vi "Get_criterion.vi"(8 "error in":errorcluster, 11 "WLAN Test Text Input":string="TX_VERIFY_EVM 5320 OFDM6 20M TX2") -> (0 "error out":errorcluster, 2 "BT_Range":T2, 3 "WLAN_Range":T1)   [LabVIEW 2012]
uses:
  <vilib>/Utility/file.llb/Read From Spreadsheet File (string).vi
panel:
  in  "MHz 2":i16=20
  out "Violation%":string
  out "row 2":i32
  out "time spend(ms)":u32
  out "Test iItem":string
  out "row":i32
  out "mode number":dbl
  out "Mode":enum16{"OFDM", "DSSS", "MCS"}(ring)
  out "column":i32
  out "Numeric":i32
  in  "MHz":i16=20
  in  "Mode string in":string="MCS7"
  out "frequency string":string
  in  "Frequency":dbl=2412000000.0 format="%#_6p"
  out "Classified Array":string[][][](array[string])
  out "Criterion array":string[][](array[string])
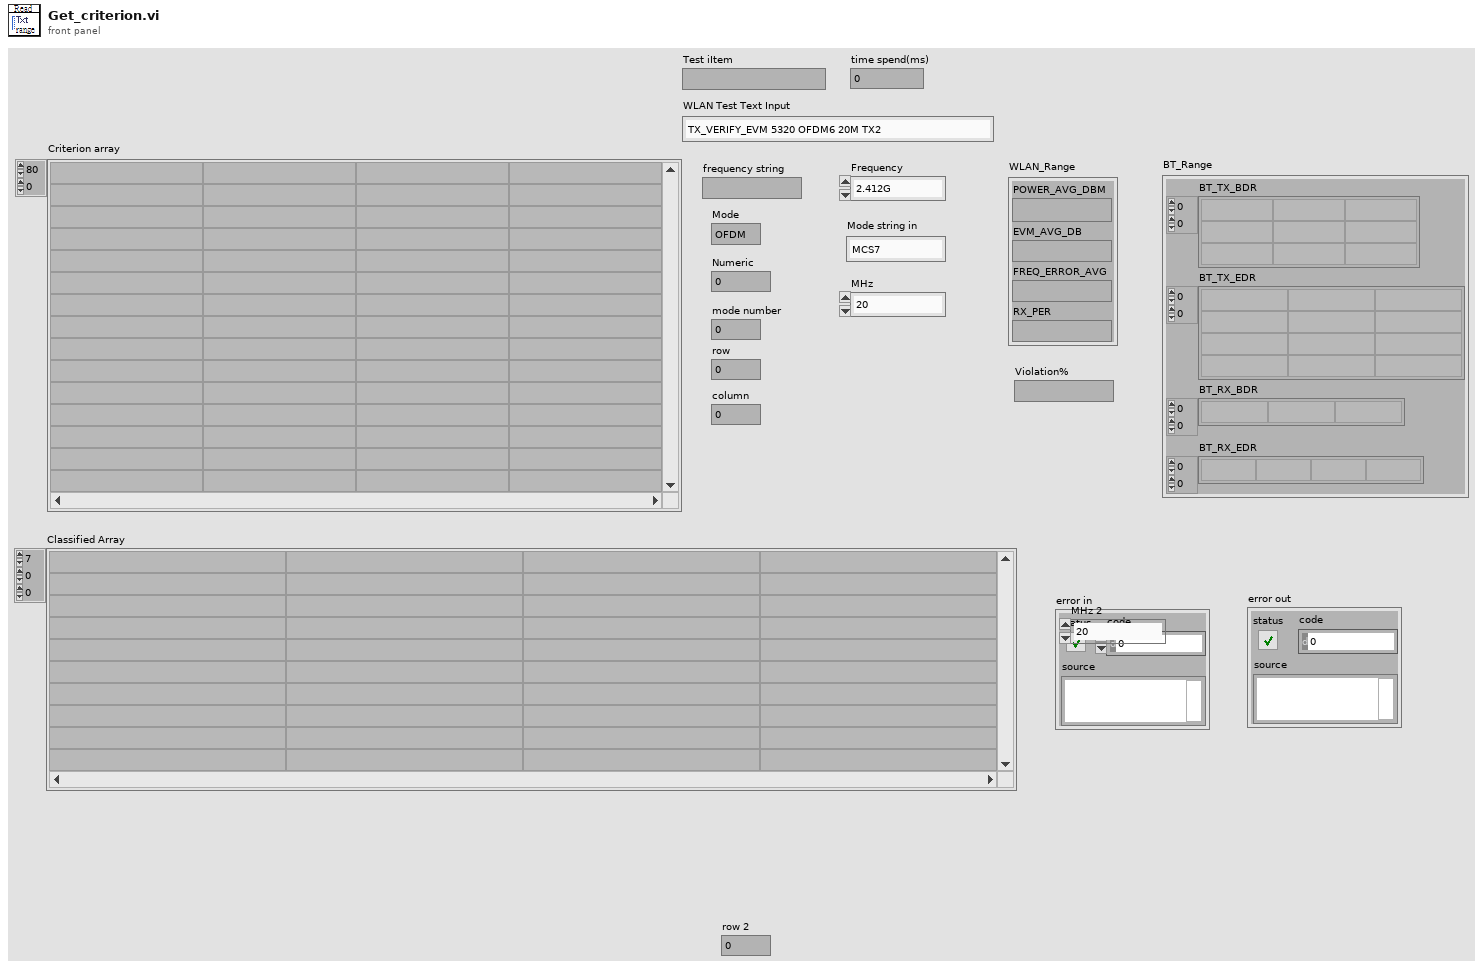
[diagram p1: front panel]
types:
  T1 = cluster{"POWER_AVG_DBM":string, "EVM_AVG_DB":string, "FREQ_ERROR_AVG":string, "RX_PER":string}
  T2 = cluster{"BT_TX_BDR":string[][], "BT_TX_EDR":string[][], "BT_RX_BDR":string[][], "BT_RX_EDR":string[][]}
  T3 = enum32{"invalid app kind", "Development System", "Run Time System", "Student Edition", "Embedded LabVIEW", "Evaluation", "Custom"}
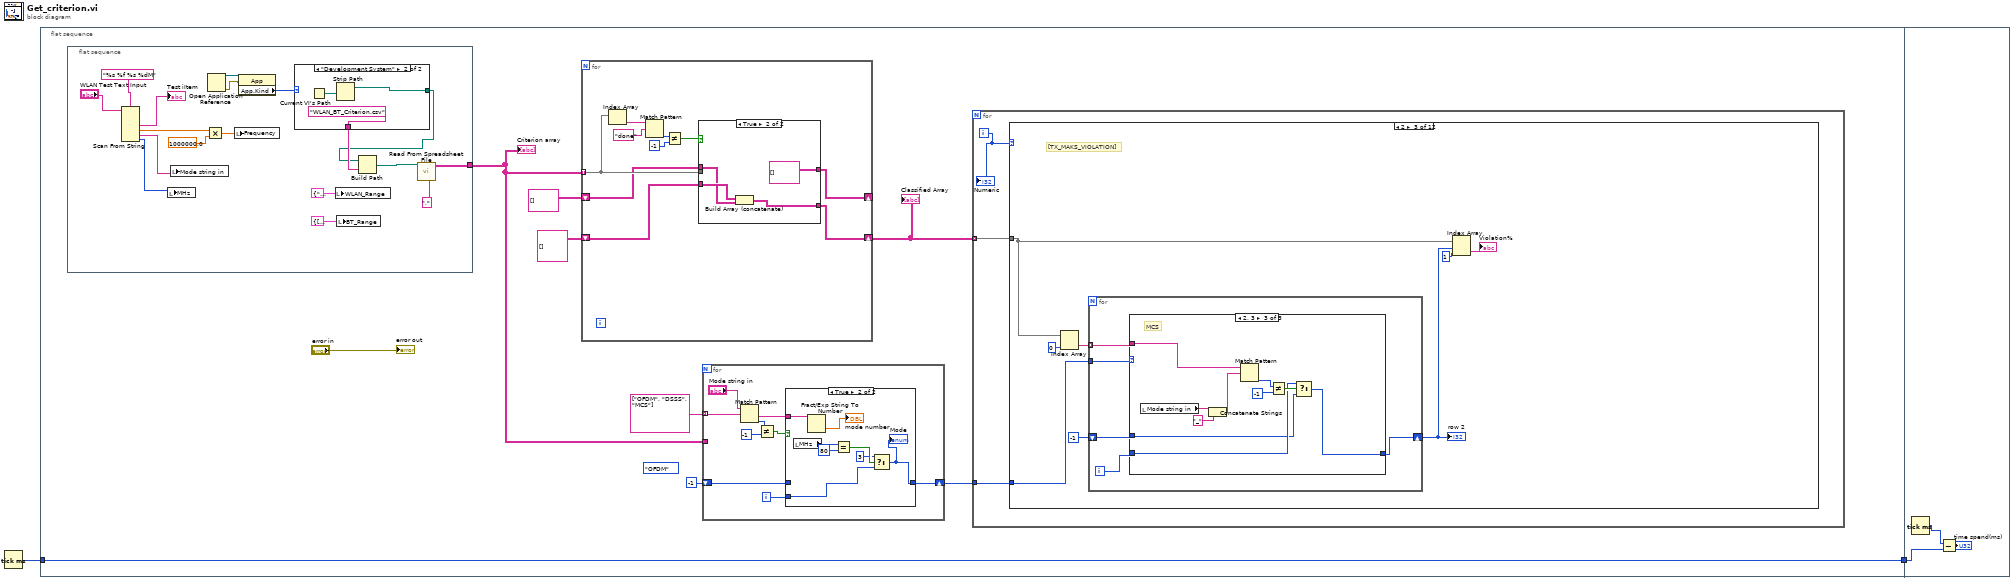
[diagram p0: block diagram]
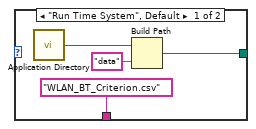
[diagram p2: hidden frame]
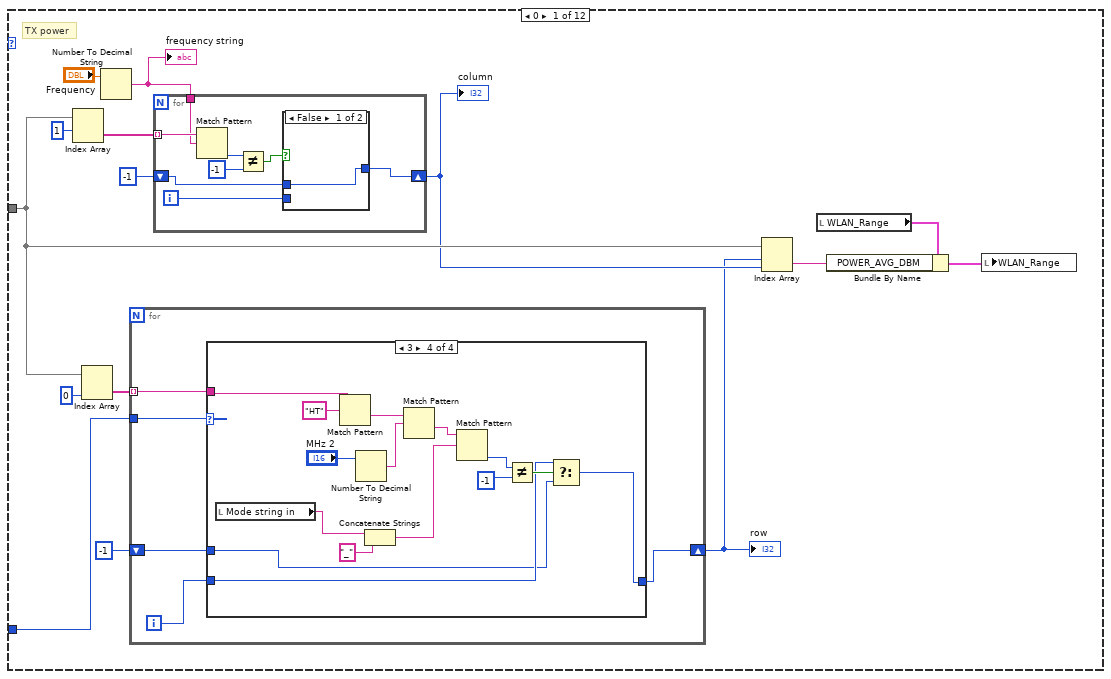
[diagram p4: hidden frame]
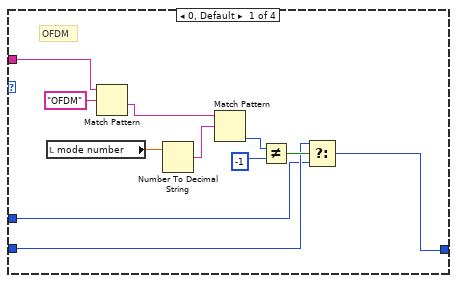
[diagram p5: hidden frame]
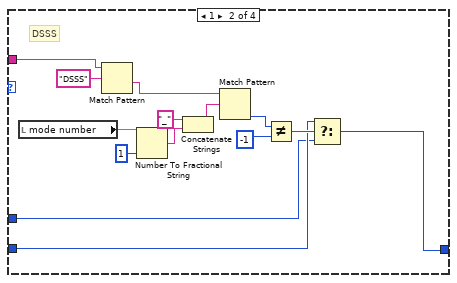
[diagram p6: hidden frame]
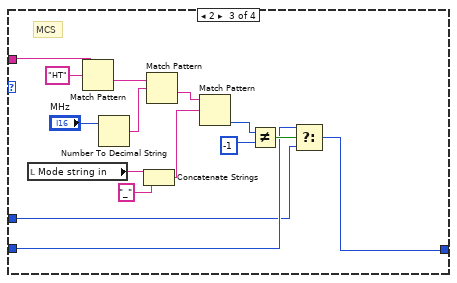
[diagram p7: hidden frame]
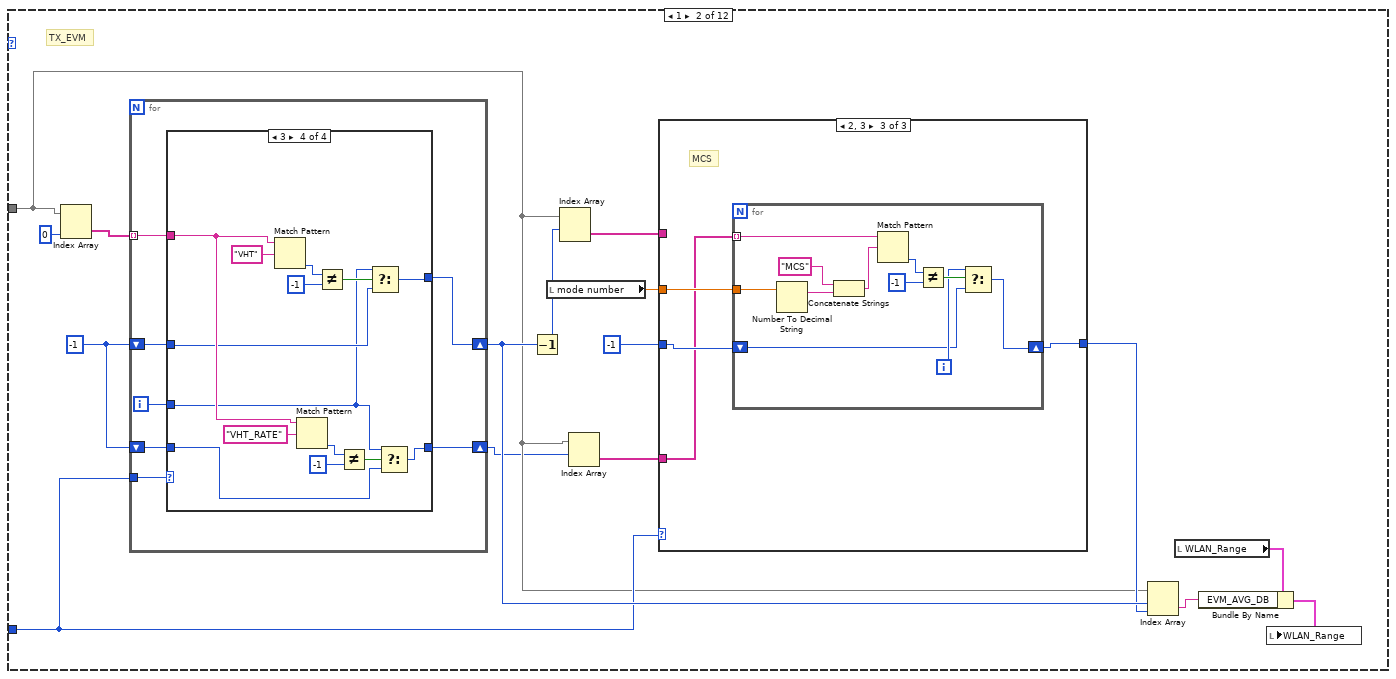
[diagram p9: hidden frame]
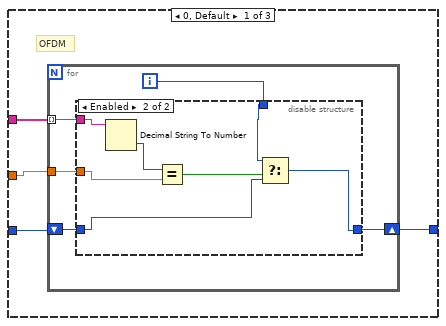
[diagram p10: hidden frame]
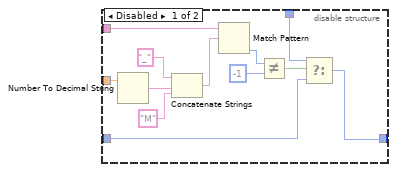
[diagram p11: hidden frame]
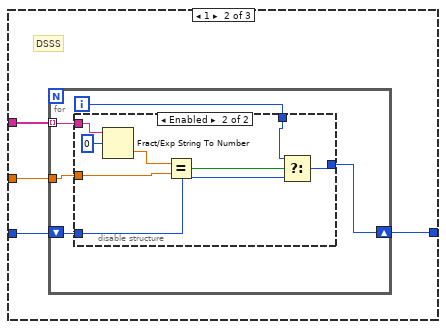
[diagram p12: hidden frame]
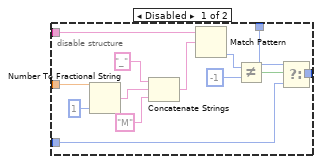
[diagram p13: hidden frame]
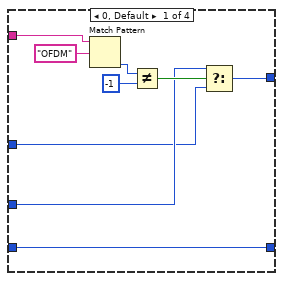
[diagram p14: hidden frame]
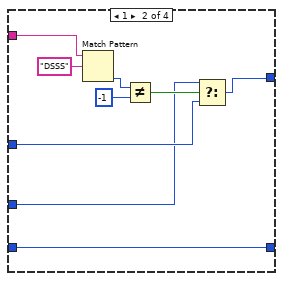
[diagram p15: hidden frame]
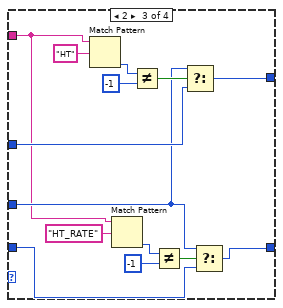
[diagram p16: hidden frame]
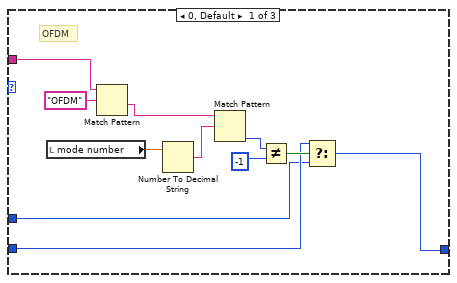
[diagram p17: hidden frame]
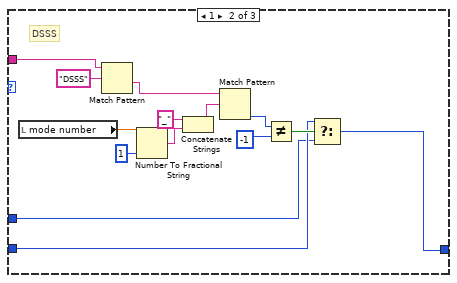
[diagram p18: hidden frame]
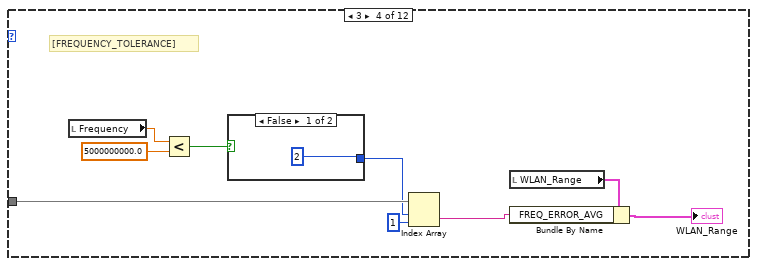
[diagram p19: hidden frame]
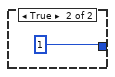
[diagram p20: hidden frame]
diagram:
  n1 = Tick Count (ms)() -> (millisecond timer value=w2:u32)
  n2 = flat-sequence {
    tunnel: w2 -> [w4]
    tunnel: [w4] -> w1
    tunnel: w1 -> [w502]
    frame #0 {
      (unwired) enum16{"OFDM", "DSSS", "MCS"}."OFDM"
      n3 = flat-sequence {
        tunnel: [w28] -> w3
        frame #0 {
          n4 = Scan From String(format string="%s %f %s %dM", input string="WLAN Test Text Input") -> (output 1=→"Test iItem":string, output 2=w21:dbl, output 3=w18:string, output 4=w17:i32)  [unwired: 6 in, 3 out]
          n5 = local write "MHz"(w17) -> ()
          n6 = local write "Mode string in"(w18) -> ()
          n7 = Multiply(x=w21, y=1000000.0) -> (x*y=w19:dbl)
          n8 = Open Application Reference() -> (0:w15:errorcluster, 3:w16:refnum<vi>)  [unwired: 4 in]
          n9 = local write "Frequency"(w19) -> ()
          n10 = property class="App"(reference=w16, error in=w15) -> ("App.Kind"=w14:T3)  [unwired: 2 out]
          n11 = case shown="\"Development System\"" w14 {
            tunnel: [w31 w35] -> w12
            tunnel: ["WLAN_BT_Criterion.csv" ("name or relative path") "WLAN_BT_Criterion.csv" ("name or relative path")] -> w13
            frame "Run Time System", Default {
              n12 = call <vilib>:"Application Directory.vi"() -> ("Application Directory"=w33:path)
              n13 = Build Path(base path=w33, name or relative path="data") -> (appended path=w31:path)
            }
            frame "Development System" {
              n14 = Current VI's Path() -> (path=w36:path)
              n15 = Strip Path(path=w36) -> (stripped path=w35:path)  [unwired: 1 out]
            }
          }
          n16 = local write "WLAN_Range"(T1 {"POWER_AVG_DBM"="", "EVM_AVG_DB"="", "FREQ_ERROR_AVG"="", "RX_PER"=""} ("WLAN_Range")) -> ()
          n17 = local write "BT_Range"(T2 {"BT_TX_BDR"=[], "BT_TX_EDR"=[], "BT_RX_BDR"=[], "BT_RX_EDR"=[]} ("BT_Range")) -> ()
          n18 = Build Path(base path=w12, name or relative path=w13) -> (appended path=w25:path)
          n19 = call-poly <vilib>:"Read From Spreadsheet File.vi"("delimiter (\\t)"="," ("delimiter (\\t)"), "file path (dialog if empty)"=w25) -> ("all rows"=w28:string[][])  [unwired: 5 in, 4 out]
        }
      }
      n20 = for {
        tunnel: w3 -> [w491] mode=indexing
        shift-right: [w489] -> _
        shift-left: string[][] [] -> [w490]
        shift-right: [w487] -> w6
        shift-left: string[][][] [] -> [w488]
        n21 = Index Array(array=w491) -> (element=w486:string)  [unwired: 1 in]
        n22 = Match Pattern(string=w486, regular expression="done") -> (offset past match=w484:i32)  [unwired: 1 in, 3 out]
        n23 = Not Equal?(x=w484, y=-1) -> (x != y?=w482:bool)
        n24 = case shown="True" w482 {
          tunnel: w490 -> [w495 w497]
          tunnel: w491 -> [w494 _]
          tunnel: [w493 string[][] []] -> w489
          tunnel: w488 -> [w492 w498]
          tunnel: [w492 w496] -> w487
          frame False {
            n25 = Build Array (concatenate)(w495, w494) -> (w493:string[][])
          }
          frame True {
            n26 = Build Array (concatenate)(w498, w497) -> (w496:string[][][])
          }
        }
      }
      "Classified Array" <- w6
      n27 = for {
        tunnel: string[] ["OFDM", "DSSS", "MCS"] -> [w44] mode=indexing
        shift-right: [w38] -> w8
        shift-left: -1 -> [w37]
        tunnel: w3 -> [_]
        i -> [w40]
        n28 = Match Pattern(string="Mode string in", regular expression=w44) -> (after substring=w39:string, offset past match=w43:i32)  [unwired: 1 in, 2 out]
        n29 = Not Equal?(x=w43, y=-1) -> (x != y?=w41:bool)
        n30 = case shown="True" w41 {
          tunnel: w40 -> [_ w48]
          tunnel: w39 -> [_ w54]
          tunnel: [w46 w47] -> w38
          tunnel: w37 -> [w46 _]
          frame False {
          }
          frame True {
            n31 = local read "MHz"() -> (w52:i16)
            n32 = Fract/Exp String To Number(string=w54) -> (number=→"mode number":dbl)  [unwired: 3 in, 1 out]
            n33 = Equal?(x=w52, y=i16 80) -> (x = y?=w50:bool)
            n34 = Select(t=3, s=w50, f=w48) -> (s? t:f=w47:i32)
            "Mode" <- w47
          }
        }
      }
      n35 = for {
        tunnel: w6 -> [w56] mode=indexing
        tunnel: w8 -> [w55]
        i -> [w57]
        n36 = case shown="2" w57 {
          tunnel: w56 -> [w63 w148 w288 w338 w349 _ _ w390 w413 w437 w461 _]
          tunnel: w55 -> [w65 w152 w289 _ w351 _ _ _ _ _ _ _]
          frame 0 {
            # "TX power"
            n37 = Index Array(array=w63, index (row)=1) -> (element=w70:string[])  [unwired: 1 in]
            n38 = Index Array(array=w63, index (col)=0) -> (element=w66:string[])  [unwired: 1 in]
            n39 = Number To Decimal String(number="Frequency") -> (decimal integer string=w69:string)  [unwired: 1 in]
            "frequency string" <- w69
            n40 = for {
              tunnel: w66 -> [w75] mode=indexing
              tunnel: w65 -> [w77]
              shift-right: [w74] -> w61
              shift-left: -1 -> [w73]
              i -> [w76]
              n41 = case shown="3" w77 {
                tunnel: w76 -> [w80 w94 w105 w120]
                tunnel: w75 -> [w87 w97 w116 w124]
                tunnel: [w79 w92 w103 w118] -> w74
                tunnel: w73 -> [w78 w93 w104 w119]
                frame 0, Default {
                  # "OFDM"
                  n42 = local read "mode number"() -> (w85:dbl)
                  n43 = Match Pattern(string=w87, regular expression="OFDM") -> (after substring=w86:string)  [unwired: 1 in, 3 out]
                  n44 = Number To Decimal String(number=w85) -> (decimal integer string=w84:string)  [unwired: 1 in]
                  n45 = Match Pattern(string=w86, regular expression=w84) -> (offset past match=w83:i32)  [unwired: 1 in, 3 out]
                  n46 = Not Equal?(x=w83, y=-1) -> (x != y?=w81:bool)
                  n47 = Select(t=w80, s=w81, f=w78) -> (s? t:f=w79:i32)
                }
                frame 1 {
                  # "DSSS"
                  n48 = local read "mode number"() -> (w96:dbl)
                  n49 = Match Pattern(string=w97, regular expression="DSSS") -> (after substring=w101:string)  [unwired: 1 in, 3 out]
                  n50 = Number To Fractional String(number=w96, precision (6)=i16 1) -> (F-format string=w90:string)  [unwired: 2 in]
                  n51 = Concatenate Strings("_" ("string"), w90) -> (w91:string)
                  n52 = Match Pattern(string=w101, regular expression=w91) -> (offset past match=w100:i32)  [unwired: 1 in, 3 out]
                  n53 = Not Equal?(x=w100, y=-1) -> (x != y?=w98:bool)
                  n54 = Select(t=w94, s=w98, f=w93) -> (s? t:f=w92:i32)
                }
                frame 2 {
                  # "MCS"
                  n55 = local read "Mode string in"() -> (w111:string)
                  n56 = Match Pattern(string=w116, regular expression="HT") -> (after substring=w114:string)  [unwired: 1 in, 3 out]
                  n57 = Number To Decimal String(number="MHz") -> (decimal integer string=w113:string)  [unwired: 1 in]
                  n58 = Concatenate Strings(w111, "_" ("string")) -> (w109:string)
                  n59 = Match Pattern(string=w114, regular expression=w113) -> (after substring=w112:string)  [unwired: 1 in, 3 out]
                  n60 = Match Pattern(string=w112, regular expression=w109) -> (offset past match=w107:i32)  [unwired: 1 in, 3 out]
                  n61 = Not Equal?(x=w107, y=-1) -> (x != y?=w106:bool)
                  n62 = Select(t=w105, s=w106, f=w104) -> (s? t:f=w103:i32)
                }
                frame 3 {
                  n63 = local read "Mode string in"() -> (w122:string)
                  n64 = Match Pattern(string=w124, regular expression="HT") -> (after substring=w130:string)  [unwired: 1 in, 3 out]
                  n65 = Number To Decimal String(number="MHz 2") -> (decimal integer string=w129:string)  [unwired: 1 in]
                  n66 = Concatenate Strings(w122, "_" ("string")) -> (w121:string)
                  n67 = Match Pattern(string=w130, regular expression=w129) -> (after substring=w128:string)  [unwired: 1 in, 3 out]
                  n68 = Match Pattern(string=w128, regular expression=w121) -> (offset past match=w126:i32)  [unwired: 1 in, 3 out]
                  n69 = Not Equal?(x=w126, y=-1) -> (x != y?=w125:bool)
                  n70 = Select(t=w120, s=w125, f=w119) -> (s? t:f=w118:i32)
                }
              }
            }
            "row" <- w61
            n71 = for {
              tunnel: w70 -> [w140] mode=indexing
              tunnel: w69 -> [w139]
              shift-right: [w134] -> w62
              shift-left: -1 -> [w133]
              i -> [w135]
              n72 = Match Pattern(string=w140, regular expression=w139) -> (offset past match=w138:i32)  [unwired: 1 in, 3 out]
              n73 = Not Equal?(x=w138, y=-1) -> (x != y?=w136:bool)
              n74 = case shown="False" w136 {
                tunnel: w135 -> [_ w142]
                tunnel: [w141 w142] -> w134
                tunnel: w133 -> [w141 _]
                frame False {
                }
                frame True {
                }
              }
            }
            "column" <- w62
            n75 = Index Array(array=w63, index (row)=w61, index (col)=w62) -> (element=w59:string)
            n76 = local read "WLAN_Range"() -> (w58:T1)
            n77 = Bundle By Name(cluster=w58, "POWER_AVG_DBM"=w59) -> (w60:T1)
            n78 = local write "WLAN_Range"(w60) -> ()
          }
          frame 1 {
            w149 = -1
            # "TX_EVM"
            n79 = Index Array(array=w148, index (col)=0) -> (element=w157:string[])  [unwired: 1 in]
            n80 = for {
              tunnel: w157 -> [w237] mode=indexing
              tunnel: w152 -> [w238]
              shift-right: [w234] -> w154
              shift-left: w149 -> [w235]
              shift-right: [w232] -> w147
              shift-left: w149 -> [w233]
              i -> [w236]
              n81 = case shown="3" w238 {
                tunnel: w237 -> [w246 w253 w257 w276]
                tunnel: w236 -> [w242 w250 w260 w274]
                tunnel: w235 -> [w241 w251 w266 w275]
                tunnel: [w240 w249 w265 w272] -> w234
                tunnel: w233 -> [w239 w248 w259 w273]
                tunnel: [w239 w248 w258 w271] -> w232
                frame 0, Default {
                  n82 = Match Pattern(string=w246, regular expression="OFDM") -> (offset past match=w245:i32)  [unwired: 1 in, 3 out]
                  n83 = Not Equal?(x=w245, y=-1) -> (x != y?=w243:bool)
                  n84 = Select(t=w242, s=w243, f=w241) -> (s? t:f=w240:i32)
                }
                frame 1 {
                  n85 = Match Pattern(string=w253, regular expression="DSSS") -> (offset past match=w256:i32)  [unwired: 1 in, 3 out]
                  n86 = Not Equal?(x=w256, y=-1) -> (x != y?=w254:bool)
                  n87 = Select(t=w250, s=w254, f=w251) -> (s? t:f=w249:i32)
                }
                frame 2 {
                  n88 = Match Pattern(string=w257, regular expression="HT") -> (offset past match=w269:i32)  [unwired: 1 in, 3 out]
                  n89 = Match Pattern(string=w257, regular expression="HT_RATE") -> (offset past match=w262:i32)  [unwired: 1 in, 3 out]
                  n90 = Not Equal?(x=w269, y=-1) -> (x != y?=w267:bool)
                  n91 = Not Equal?(x=w262, y=-1) -> (x != y?=w264:bool)
                  n92 = Select(t=w260, s=w267, f=w266) -> (s? t:f=w265:i32)
                  n93 = Select(t=w260, s=w264, f=w259) -> (s? t:f=w258:i32)
                }
                frame 3 {
                  n94 = Match Pattern(string=w276, regular expression="VHT") -> (offset past match=w283:i32)  [unwired: 1 in, 3 out]
                  n95 = Match Pattern(string=w276, regular expression="VHT_RATE") -> (offset past match=w278:i32)  [unwired: 1 in, 3 out]
                  n96 = Not Equal?(x=w283, y=-1) -> (x != y?=w281:bool)
                  n97 = Not Equal?(x=w278, y=-1) -> (x != y?=w280:bool)
                  n98 = Select(t=w274, s=w281, f=w275) -> (s? t:f=w272:i32)
                  n99 = Select(t=w274, s=w280, f=w273) -> (s? t:f=w271:i32)
                }
              }
            }
            n100 = Decrement(x=w154) -> (x-1=w156:i32)
            n101 = local read "mode number"() -> (w151:dbl)
            n102 = Index Array(array=w148, index (row)=w156) -> (element=w155:string[])  [unwired: 1 in]
            n103 = Index Array(array=w148, index (row)=w147) -> (element=w146:string[])  [unwired: 1 in]
            n104 = case shown="2, 3" w152 {
              tunnel: w155 -> [w162 w190 _]
              tunnel: [w161 w189 w217] -> w153
              tunnel: w151 -> [w160 w188 w219]
              tunnel: -1 -> [w159 w187 w220]
              tunnel: w146 -> [_ _ w218]
              frame 0, Default {
                # "OFDM"
                n105 = for {
                  tunnel: w162 -> [w167] mode=indexing
                  shift-right: [w164] -> w161
                  shift-left: w159 -> [w165]
                  tunnel: w160 -> [w163]
                  i -> [w166]
                  n106 = disable-structure shown="Enabled" {
                    disable-tunnel: w167 -> [w179 w186]
                    disable-tunnel: w166 -> [w178 w182]
                    disable-tunnel: w165 -> [w177 w181]
                    disable-tunnel: [w176 w180] -> w164
                    disable-tunnel: w163 -> [w175 w184]
                    frame Disabled {
                      n107 = Number To Decimal String(number=w175) -> (decimal integer string=w171:string)  [unwired: 1 in]
                      n108 = Concatenate Strings("_" ("string"), w171, "M" ("string")) -> (w168:string)
                      n109 = Match Pattern(string=w179, regular expression=w168) -> (offset past match=w173:i32)  [unwired: 1 in, 3 out]
                      n110 = Not Equal?(x=w173, y=-1) -> (x != y?=w172:bool)
                      n111 = Select(t=w178, s=w172, f=w177) -> (s? t:f=w176:i32)
                    }
                    frame Enabled {
                      n112 = Decimal String To Number(string=w186) -> (number=w185:i32)  [unwired: 2 in, 1 out]
                      n113 = Equal?(x=w185, y=w184) -> (x = y?=w183:bool)
                      n114 = Select(t=w182, s=w183, f=w181) -> (s? t:f=w180:i32)
                    }
                  }
                }
              }
              frame 1 {
                # "DSSS"
                n115 = for {
                  tunnel: w190 -> [w195] mode=indexing
                  shift-right: [w192] -> w189
                  shift-left: w187 -> [w193]
                  tunnel: w188 -> [w191]
                  i -> [w194]
                  n116 = disable-structure shown="Enabled" {
                    disable-tunnel: w195 -> [w208 w216]
                    disable-tunnel: w194 -> [w204 w212]
                    disable-tunnel: w193 -> [w203 w211]
                    disable-tunnel: [w202 w210] -> w192
                    disable-tunnel: w191 -> [w196 w214]
                    frame Disabled {
                      n117 = Number To Fractional String(number=w196, precision (6)=i16 1) -> (F-format string=w197:string)  [unwired: 2 in]
                      n118 = Concatenate Strings("_" ("string"), w197, "M" ("string")) -> (w199:string)
                      n119 = Match Pattern(string=w208, regular expression=w199) -> (offset past match=w206:i32)  [unwired: 1 in, 3 out]
                      n120 = Not Equal?(x=w206, y=-1) -> (x != y?=w205:bool)
                      n121 = Select(t=w204, s=w205, f=w203) -> (s? t:f=w202:i32)
                    }
                    frame Enabled {
                      n122 = Fract/Exp String To Number(string=w216, offset=0) -> (number=w215:dbl)  [unwired: 2 in, 1 out]
                      n123 = Equal?(x=w215, y=w214) -> (x = y?=w213:bool)
                      n124 = Select(t=w212, s=w213, f=w211) -> (s? t:f=w210:i32)
                    }
                  }
                }
              }
              frame 2, 3 {
                # "MCS"
                n125 = for {
                  tunnel: w218 -> [w231] mode=indexing
                  shift-right: [w225] -> w217
                  shift-left: w220 -> [w226]
                  tunnel: w219 -> [w221]
                  i -> [w227]
                  n126 = Number To Decimal String(number=w221) -> (decimal integer string=w224:string)  [unwired: 1 in]
                  n127 = Concatenate Strings("MCS" ("string"), w224) -> (w222:string)
                  n128 = Match Pattern(string=w231, regular expression=w222) -> (offset past match=w229:i32)  [unwired: 1 in, 3 out]
                  n129 = Not Equal?(x=w229, y=-1) -> (x != y?=w228:bool)
                  n130 = Select(t=w227, s=w228, f=w226) -> (s? t:f=w225:i32)
                }
              }
            }
            n131 = Index Array(array=w148, index (row)=w154, index (col)=w153) -> (element=w145:string)
            n132 = local read "WLAN_Range"() -> (w143:T1)
            n133 = Bundle By Name(cluster=w143, "EVM_AVG_DB"=w145) -> (w144:T1)
            n134 = local write "WLAN_Range"(w144) -> ()
          }
          frame 2 {
            # "[TX_MAKS_VIOLATION]"
            n135 = Index Array(array=w288, index (col)=0) -> (element=w291:string[])  [unwired: 1 in]
            n136 = for {
              tunnel: w291 -> [w296] mode=indexing
              tunnel: w289 -> [w295]
              shift-right: [w297] -> w287
              shift-left: -1 -> [w294]
              i -> [w293]
              n137 = case shown="2, 3" w295 {
                tunnel: w293 -> [w300 w314 w326]
                tunnel: w296 -> [w307 w317 w323]
                tunnel: [w299 w312 w324] -> w297
                tunnel: w294 -> [w298 w313 w325]
                frame 0, Default {
                  # "OFDM"
                  n138 = local read "mode number"() -> (w305:dbl)
                  n139 = Match Pattern(string=w307, regular expression="OFDM") -> (after substring=w306:string)  [unwired: 1 in, 3 out]
                  n140 = Number To Decimal String(number=w305) -> (decimal integer string=w304:string)  [unwired: 1 in]
                  n141 = Match Pattern(string=w306, regular expression=w304) -> (offset past match=w303:i32)  [unwired: 1 in, 3 out]
                  n142 = Not Equal?(x=w303, y=-1) -> (x != y?=w301:bool)
                  n143 = Select(t=w300, s=w301, f=w298) -> (s? t:f=w299:i32)
                }
                frame 1 {
                  # "DSSS"
                  n144 = local read "mode number"() -> (w316:dbl)
                  n145 = Match Pattern(string=w317, regular expression="DSSS") -> (after substring=w321:string)  [unwired: 1 in, 3 out]
                  n146 = Number To Fractional String(number=w316, precision (6)=i16 1) -> (F-format string=w310:string)  [unwired: 2 in]
                  n147 = Concatenate Strings("_" ("string"), w310) -> (w311:string)
                  n148 = Match Pattern(string=w321, regular expression=w311) -> (offset past match=w320:i32)  [unwired: 1 in, 3 out]
                  n149 = Not Equal?(x=w320, y=-1) -> (x != y?=w318:bool)
                  n150 = Select(t=w314, s=w318, f=w313) -> (s? t:f=w312:i32)
                }
                frame 2, 3 {
                  # "MCS"
                  n151 = local read "Mode string in"() -> (w332:string)
                  n152 = Concatenate Strings(w332, "_" ("string")) -> (w330:string)
                  n153 = Match Pattern(string=w323, regular expression=w330) -> (offset past match=w328:i32)  [unwired: 1 in, 3 out]
                  n154 = Not Equal?(x=w328, y=-1) -> (x != y?=w327:bool)
                  n155 = Select(t=w326, s=w327, f=w325) -> (s? t:f=w324:i32)
                }
              }
            }
            "row 2" <- w287
            n156 = Index Array(array=w288, index (row)=w287, index (col)=1 ("disabled index (col)")) -> (element=→"Violation%":string)
          }
          frame 3 {
            # "[FREQUENCY_TOLERANCE]"
            n157 = local read "Frequency"() -> (w341:dbl)
            n158 = Less?(x=w341, y=5000000000.0) -> (x < y?=w339:bool)
            n159 = case shown="False" w339 {
              tunnel: [2 1] -> w336
              frame False {
              }
              frame True {
              }
            }
            n160 = Index Array(array=w338, index (row)=w336, index (col)=1 ("disabled index (col)")) -> (element=w335:string)
            n161 = local read "WLAN_Range"() -> (w333:T1)
            n162 = Bundle By Name(cluster=w333, "FREQ_ERROR_AVG"=w335) -> (→"WLAN_Range":T1)
          }
          frame 4 {
            # "[RX_PER]"
            n163 = Index Array(array=w349, index (col)=0 ("disabled index (col)")) -> (element=w352:string[])  [unwired: 1 in]
            n164 = for {
              tunnel: w352 -> [w357] mode=indexing
              tunnel: w351 -> [w358]
              shift-right: [w354] -> w347
              shift-left: -1 ("y") -> [w356]
              i -> [w355]
              n165 = case shown="0, Default" w358 {
                tunnel: w357 -> [w366 w371 w384]
                tunnel: w356 -> [w361 w369 w377]
                tunnel: w355 -> [w360 w368 w376]
                tunnel: [w359 w367 w375] -> w354
                frame 0, Default {
                  n166 = Match Pattern(string=w366, regular expression="OFDM") -> (offset past match=w363:i32)  [unwired: 1 in, 3 out]
                  n167 = Not Equal?(x=w363, y=-1) -> (x != y?=w362:bool)
                  n168 = Select(t=w360, s=w362, f=w361) -> (s? t:f=w359:i32)
                }
                frame 1 {
                  n169 = Match Pattern(string=w371, regular expression="DSSS") -> (offset past match=w372:i32)  [unwired: 1 in, 3 out]
                  n170 = Not Equal?(x=w372, y=-1) -> (x != y?=w370:bool)
                  n171 = Select(t=w368, s=w370, f=w369) -> (s? t:f=w367:i32)
                }
                frame 2 {
                  n172 = local read "MHz"() -> (w382:i16)
                  n173 = Match Pattern(string=w384, regular expression="HT") -> (after substring=w383:string)  [unwired: 1 in, 3 out]
                  n174 = Number To Decimal String(number=w382) -> (decimal integer string=w381:string)  [unwired: 1 in]
                  n175 = Match Pattern(string=w383, regular expression=w381) -> (offset past match=w380:i32)  [unwired: 1 in, 3 out]
                  n176 = Not Equal?(x=w380, y=-1) -> (x != y?=w378:bool)
                  n177 = Select(t=w376, s=w378, f=w377) -> (s? t:f=w375:i32)
                }
              }
            }
            n178 = Index Array(array=w349, index (row)=w347, index (col)=1 ("index (row)")) -> (element=w345:string)
            n179 = local read "WLAN_Range"() -> (w344:T1)
            n180 = Bundle By Name(cluster=w344, "RX_PER"=w345) -> (w346:T1)
            n181 = local write "WLAN_Range"(w346) -> ()
          }
          frame 5 {
            # "[RX_SENSITIVITY_START_SEARCH_POW"
          }
          frame 6 {
            # "[RX_SENSITIVITY]"
          }
          frame 7 {
            # "[BT_TX_BDR]"
            n182 = for {
              tunnel: w390 -> [w398] mode=indexing
              shift-right: [w396] -> w387
              shift-left: string[][] [] -> [w397]
              w399 = ""
              n183 = Index Array(array=w398, index #1=0 ("index"), index #2=1 ("index"), index #3=2 ("index")) -> (element #1=w402:string, element #2=w401:string, element #3=w400:string)
              n184 = Not Equal?(x=w402, y=w399) -> (x != y?=w394:bool)
              n185 = Not Equal?(x=w401, y=w399) -> (x != y?=w392:bool)
              n186 = Not Equal?(x=w400, y=w399) -> (x != y?=w393:bool)
              n187 = Or(x=w392, y=w393) -> (x .or. y?=w391:bool)
              n188 = And(x=w394, y=w391) -> (x .and. y?=w395:bool)
              n189 = case shown="True" w395 {
                tunnel: w398 -> [_ w408]
                tunnel: w397 -> [w406 w409]
                tunnel: [w406 w407] -> w396
                frame False {
                }
                frame True {
                  n190 = Build Array (concatenate)(w409, w408) -> (w407:string[][])
                }
              }
            }
            n191 = local read "BT_Range"() -> (w386:T2)
            n192 = Bundle By Name(cluster=w386, "BT_TX_BDR"=w387) -> (w388:T2)
            n193 = local write "BT_Range"(w388) -> ()
          }
          frame 8 {
            # "[BT_TX_EDR]"
            n194 = for {
              tunnel: w413 -> [w422] mode=indexing
              shift-right: [w420] -> w411
              shift-left: string[][] [] -> [w421]
              w423 = ""
              n195 = Index Array(array=w422, index #1=0 ("index"), index #2=1 ("index"), index #3=2 ("index")) -> (element #1=w426:string, element #2=w425:string, element #3=w424:string)
              n196 = Not Equal?(x=w426, y=w423) -> (x != y?=w418:bool)
              n197 = Not Equal?(x=w425, y=w423) -> (x != y?=w416:bool)
              n198 = Not Equal?(x=w424, y=w423) -> (x != y?=w417:bool)
              n199 = Or(x=w416, y=w417) -> (x .or. y?=w415:bool)
              n200 = And(x=w418, y=w415) -> (x .and. y?=w419:bool)
              n201 = case shown="False" w419 {
                tunnel: w422 -> [_ w432]
                tunnel: w421 -> [w430 w433]
                tunnel: [w430 w431] -> w420
                frame False {
                }
                frame True {
                  n202 = Build Array (concatenate)(w433, w432) -> (w431:string[][])
                }
              }
            }
            n203 = local read "BT_Range"() -> (w410:T2)
            n204 = Bundle By Name(cluster=w410, "BT_TX_EDR"=w411) -> (w412:T2)
            n205 = local write "BT_Range"(w412) -> ()
          }
          frame 9 {
            # "[BT_RX_BDR]"
            n206 = for {
              tunnel: w437 -> [w446] mode=indexing
              shift-right: [w444] -> w435
              shift-left: string[][] [] -> [w445]
              w447 = ""
              n207 = Index Array(array=w446, index #1=0 ("index"), index #2=1 ("index"), index #3=2 ("index")) -> (element #1=w450:string, element #2=w449:string, element #3=w448:string)
              n208 = Not Equal?(x=w450, y=w447) -> (x != y?=w442:bool)
              n209 = Not Equal?(x=w449, y=w447) -> (x != y?=w440:bool)
              n210 = Not Equal?(x=w448, y=w447) -> (x != y?=w441:bool)
              n211 = Or(x=w440, y=w441) -> (x .or. y?=w439:bool)
              n212 = And(x=w442, y=w439) -> (x .and. y?=w443:bool)
              n213 = case shown="False" w443 {
                tunnel: w446 -> [_ w456]
                tunnel: w445 -> [w454 w457]
                tunnel: [w454 w455] -> w444
                frame False {
                }
                frame True {
                  n214 = Build Array (concatenate)(w457, w456) -> (w455:string[][])
                }
              }
            }
            n215 = local read "BT_Range"() -> (w434:T2)
            n216 = Bundle By Name(cluster=w434, "BT_RX_BDR"=w435) -> (w436:T2)
            n217 = local write "BT_Range"(w436) -> ()
          }
          frame 10 {
            # "[BT_RX_EDR]"
            n218 = for {
              tunnel: w461 -> [w470] mode=indexing
              shift-right: [w468] -> w460
              shift-left: string[][] [] -> [w469]
              w471 = ""
              n219 = Index Array(array=w470, index #1=0 ("index"), index #2=1 ("index"), index #3=2 ("index")) -> (element #1=w474:string, element #2=w473:string, element #3=w472:string)
              n220 = Not Equal?(x=w474, y=w471) -> (x != y?=w466:bool)
              n221 = Not Equal?(x=w473, y=w471) -> (x != y?=w464:bool)
              n222 = Not Equal?(x=w472, y=w471) -> (x != y?=w465:bool)
              n223 = Or(x=w464, y=w465) -> (x .or. y?=w463:bool)
              n224 = And(x=w466, y=w463) -> (x .and. y?=w467:bool)
              n225 = case shown="False" w467 {
                tunnel: w470 -> [_ w480]
                tunnel: w469 -> [w478 w481]
                tunnel: [w478 w479] -> w468
                frame False {
                }
                frame True {
                  n226 = Build Array (concatenate)(w481, w480) -> (w479:string[][])
                }
              }
            }
            n227 = local read "BT_Range"() -> (w458:T2)
            n228 = Bundle By Name(cluster=w458, "BT_RX_EDR"=w460) -> (→"BT_Range":T2)
          }
          frame -1, Default {
          }
        }
        "Numeric" <- w57
      }
      "Criterion array" <- w3
      "error out" <- "error in"
    }
    frame #1 {
      n229 = Tick Count (ms)() -> (millisecond timer value=w500:u32)
      n230 = Subtract(x=w500, y=w502) -> (x-y=→"time spend(ms)":u32)
    }
  }
